vi "Profiler.vi"(8 "error in":errorcluster, 10 "Step array":T1, 11 "Step number":i32) -> (0 "error out":errorcluster, 2 "Step number":i32, 3 "Step name":string)   [LabVIEW 2014]
uses:
  Controls/Step array.ctl
  Step/Control/Step name enum.ctl
  Step/Step global.vi
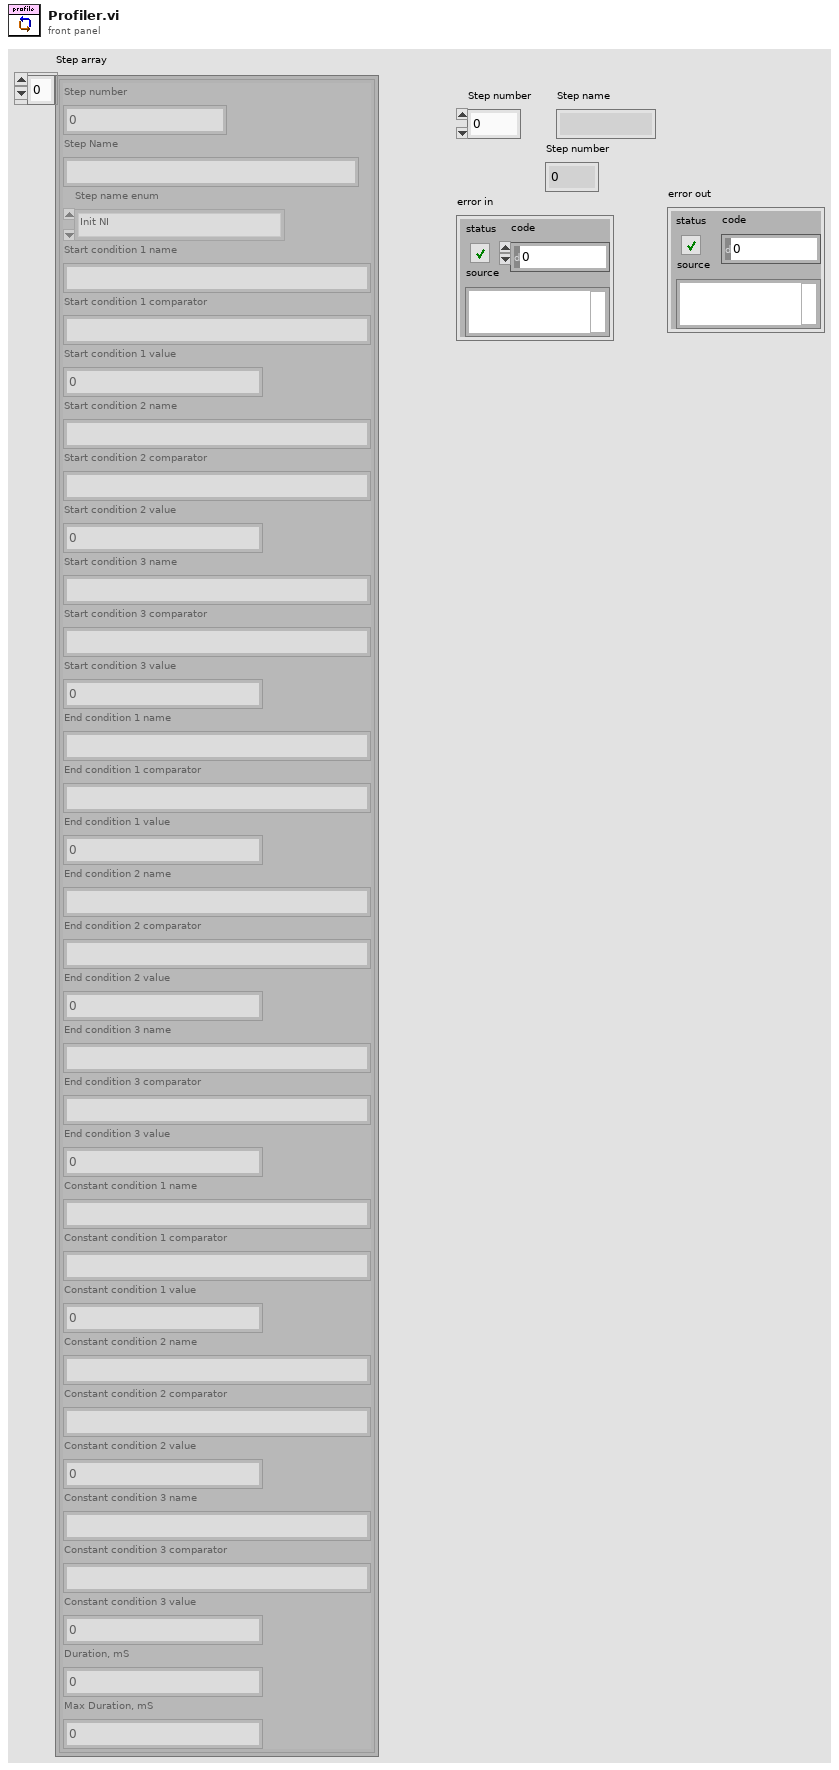
[diagram p1: front panel]
types:
  T1 = typedef "Step array.ctl" = cluster{"Step number":i32, "Step Name":string, "Step name enum":T2, "Start condition 1 name":string, "Start condition 1 comparator":string, "Start condition 1 value":dbl, "Start condition 2 name":string, "Start condition 2 comparator":string, "Start condition 2 value":dbl, "Start condition 3 name":string, "Start condition 3 comparator":string, "Start condition 3 value":dbl, "End condition 1 name":string, "End condition 1 comparator":string, "End condition 1 value":dbl, "End condition 2 name":string, "End condition 2 comparator":string, "End condition 2 value":dbl, "End condition 3 name":string, "End condition 3 comparator":string, "End condition 3 value":dbl, "Constant condition 1 name":string, "Constant condition 1 comparator":string, "Constant condition 1 value":dbl, "Constant condition 2 name":string, "Constant condition 2 comparator":string, "Constant condition 2 value":dbl, "Constant condition 3 name":string, "Constant condition 3 comparator":string, "Constant condition 3 value":dbl, "Duration, mS":dbl, "Max Duration, mS":dbl}[]
  T2 = typedef "Step name enum.ctl" = enum16{"Default", "Idle", "Init Ard", "Init SM", "Init NI", "Run", "Close"}
  T3 = cluster{"Step number":i32, "Step Name":string, "Step name enum":T2, "Start condition 1 name":string, "Start condition 1 comparator":string, "Start condition 1 value":dbl, "Start condition 2 name":string, "Start condition 2 comparator":string, "Start condition 2 value":dbl, "Start condition 3 name":string, "Start condition 3 comparator":string, "Start condition 3 value":dbl, "End condition 1 name":string, "End condition 1 comparator":string, "End condition 1 value":dbl, "End condition 2 name":string, "End condition 2 comparator":string, "End condition 2 value":dbl, "End condition 3 name":string, "End condition 3 comparator":string, "End condition 3 value":dbl, "Constant condition 1 name":string, "Constant condition 1 comparator":string, "Constant condition 1 value":dbl, "Constant condition 2 name":string, "Constant condition 2 comparator":string, "Constant condition 2 value":dbl, "Constant condition 3 name":string, "Constant condition 3 comparator":string, "Constant condition 3 value":dbl, "Duration, mS":dbl, "Max Duration, mS":dbl}
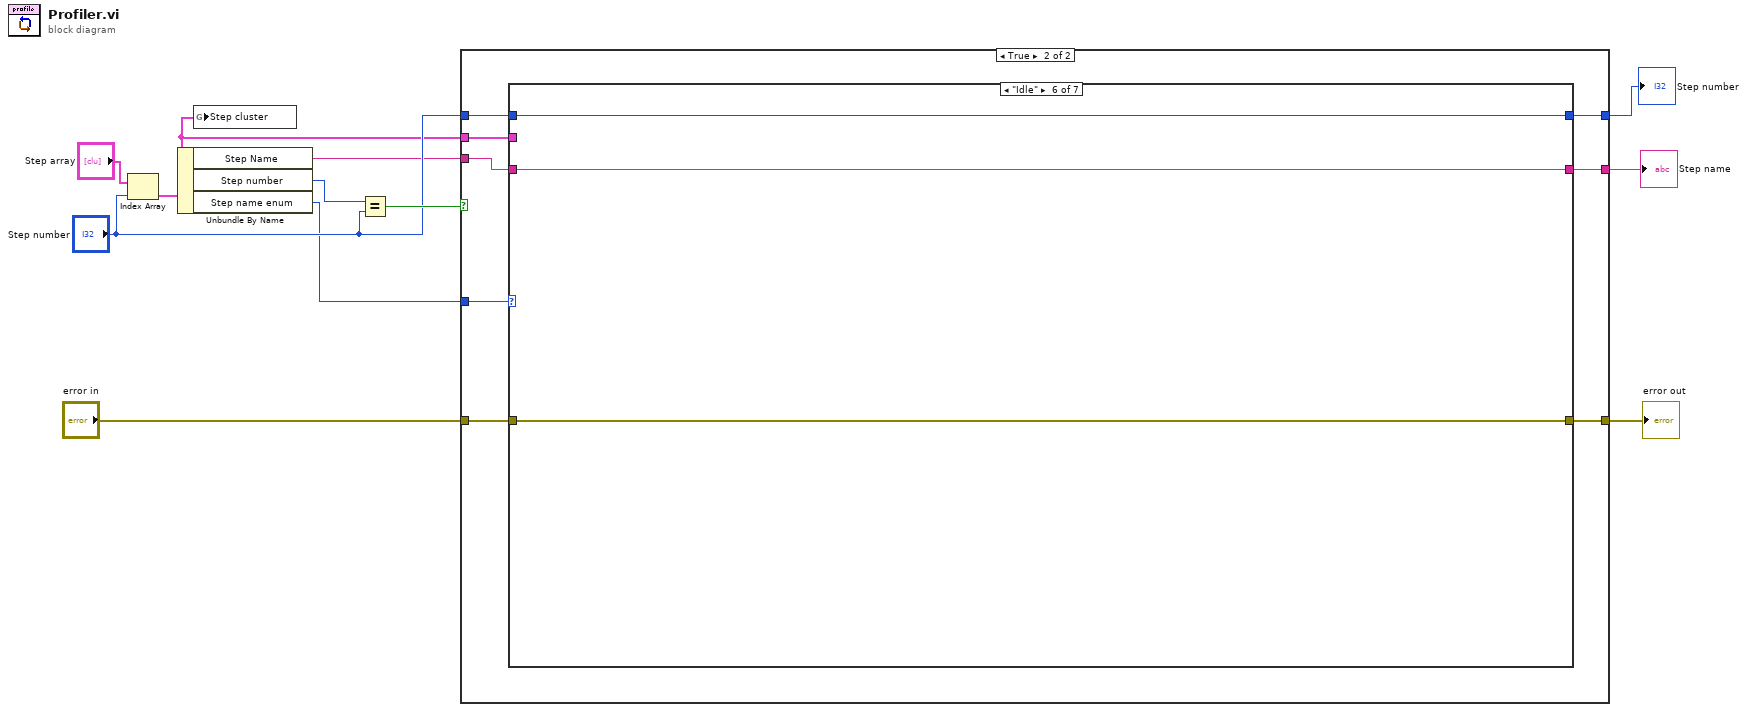
[diagram p0: block diagram]
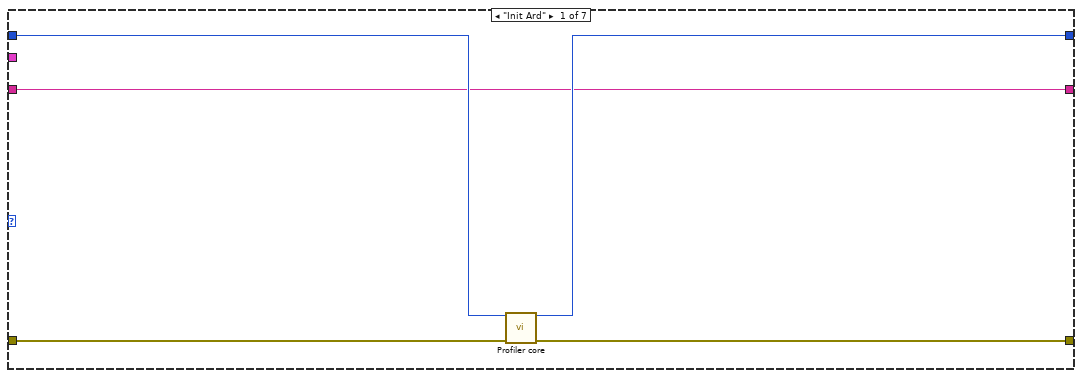
[diagram p3: hidden frame]
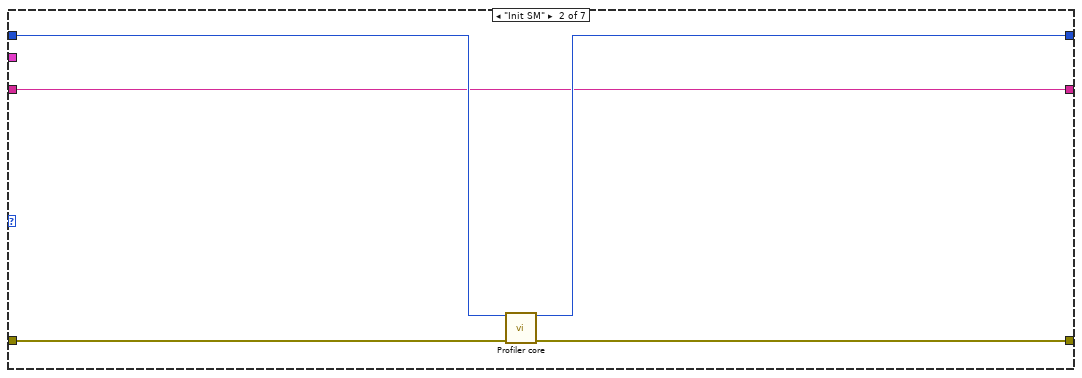
[diagram p4: hidden frame]
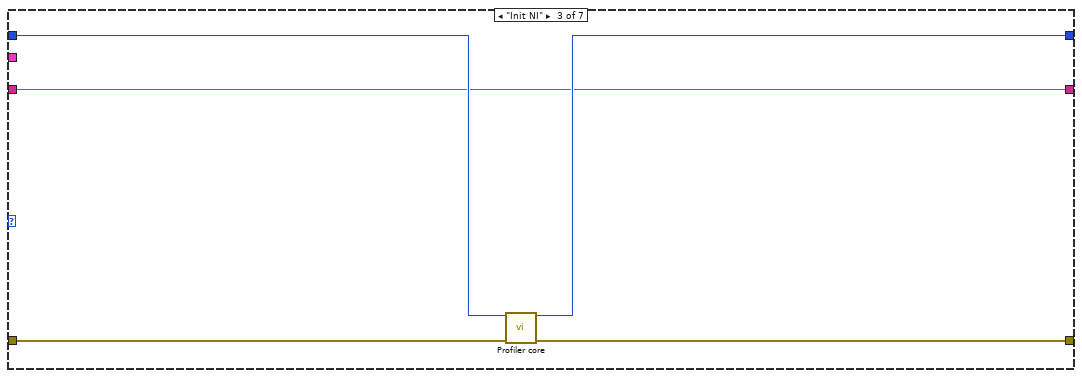
[diagram p5: hidden frame]
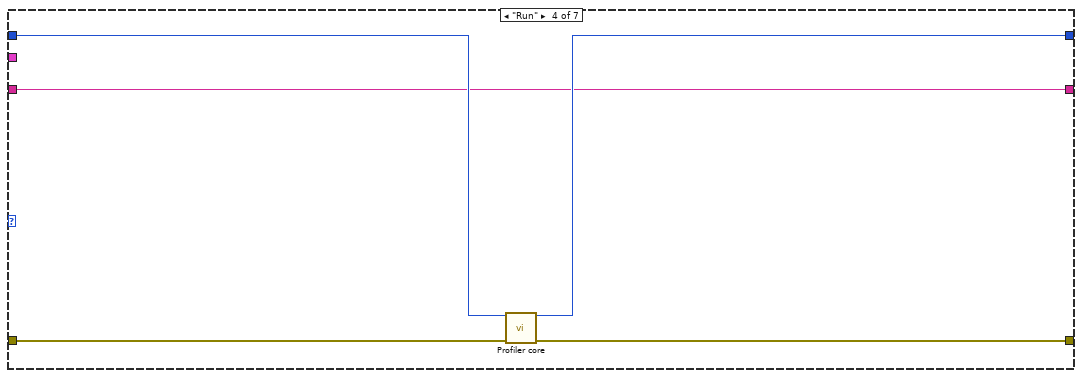
[diagram p6: hidden frame]
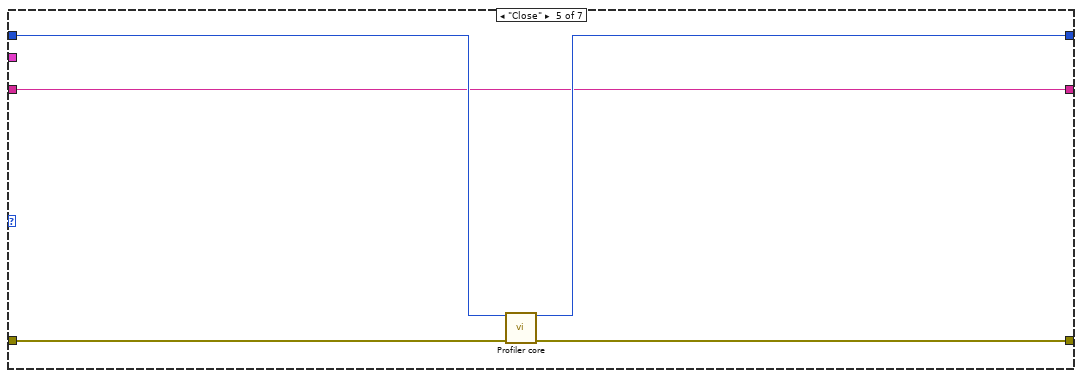
[diagram p7: hidden frame]
diagram:
  n1 = Index Array(array="Step array", index="Step number") -> (element=w3:T3)
  n2 = Unbundle By Name(w3) -> ("Step Name"=w4:string, "Step number"=w1:i32, "Step name enum"=w2:T2)
  n3 = global write "Step global.vi" "Step cluster"(w3) -> ()
  n4 = Equal?(x=w1, y="Step number") -> (x = y?=w10:bool)
  n5 = case shown="True" w10 {
    tunnel: w4 -> [w13 w16]
    tunnel: "Step number" -> [w14 w22]
    tunnel: w3 -> [_ w21]
    tunnel: [w14 w20] -> w8
    tunnel: [w13 w19] -> w7
    tunnel: "error in" -> [w12 w18]
    tunnel: [w12 w17] -> w5
    tunnel: w2 -> [_ w15]
    frame False {
    }
    frame True {
      n6 = case shown="\"Idle\"" w15 {
        tunnel: w22 -> [w25 w30 w35 w40 w45 w50 w53]
        tunnel: w21 -> [_ _ _ _ _ _ _]
        tunnel: [w24 w29 w34 w39 w44 w50 w53] -> w20
        tunnel: [w23 w28 w33 w38 w43 w49 w52] -> w19
        tunnel: w16 -> [w23 w28 w33 w38 w43 w49 w52]
        tunnel: w18 -> [w27 w32 w37 w42 w47 w48 w51]
        tunnel: [w26 w31 w36 w41 w46 w48 w51] -> w17
        frame "Init Ard" {
          n7 = call "Profiler core.vi"("Step number in"=w25, "error in"=w27) -> ("Step number out"=w24:i32, "error out"=w26:errorcluster)  [unwired: 12 in]
        }
        frame "Init SM" {
          n8 = call "Profiler core.vi"("Step number in"=w30, "error in"=w32) -> ("Step number out"=w29:i32, "error out"=w31:errorcluster)  [unwired: 12 in]
        }
        frame "Init NI" {
          n9 = call "Profiler core.vi"("Step number in"=w35, "error in"=w37) -> ("Step number out"=w34:i32, "error out"=w36:errorcluster)  [unwired: 12 in]
        }
        frame "Run" {
          n10 = call "Profiler core.vi"("Step number in"=w40, "error in"=w42) -> ("Step number out"=w39:i32, "error out"=w41:errorcluster)  [unwired: 12 in]
        }
        frame "Close" {
          n11 = call "Profiler core.vi"("Step number in"=w45, "error in"=w47) -> ("Step number out"=w44:i32, "error out"=w46:errorcluster)  [unwired: 12 in]
        }
        frame "Idle" {
        }
        frame "Default", Default {
        }
      }
    }
  }
  "Step name" <- w7
  "Step number" <- w8
  "error out" <- w5
